vi "GetStaleFilesFromDisk.vi"(8 "error in (no error)":errorcluster, 10 "BacklogBatchSize":i32, 11 "data directory":path) -> (0 "error out":errorcluster, 2 "files found":i32, 3 "file paths":path[](array[path]))   [LabVIEW 2017, in "FileManager.lvlib"]
uses:
  <vilib>/addons/InsightCM/Devices/Shared/Common/FileManager/FileManager.lvlib
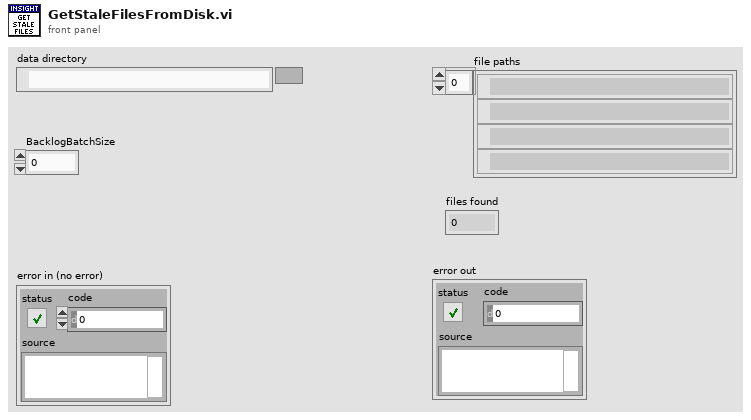
[diagram p1: front panel]
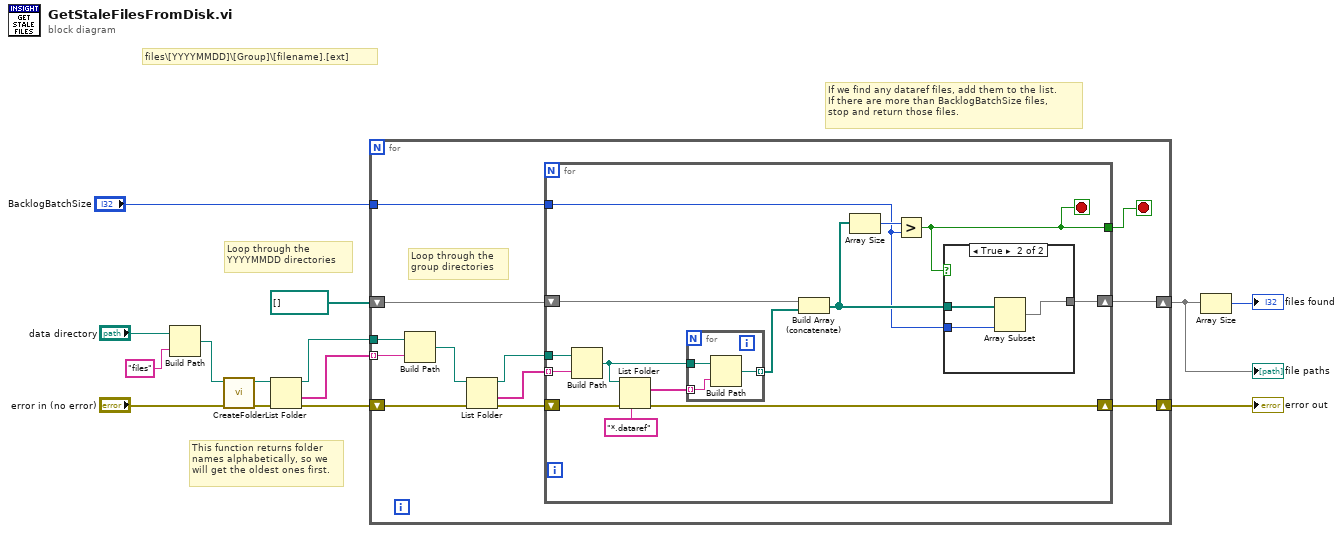
[diagram p0: block diagram]
diagram:
  # "If we find any dataref files, add them to the list.  \nIf there are more than BacklogBatchSize files,\nstop and return those files."
  # "files\\[YYYYMMDD]\\[Group]\\[filename].[ext]"
  # "This function returns folder\nnames alphabetically, so we \nwill get the oldest ones first."
  # "Loop through the \nYYYYMMDD directories"
  n1 = Build Path(base path="data directory", name or relative path="files") -> (appended path=w13:path)
  n2 = call <vilib>:"CreateFolder.vi"("error in (no error)"="error in (no error)", "folder"=w13) -> ("error out"=w10:errorcluster, "folder out"=w11:path)  [unwired: 8 in]
  n3 = List Folder(path=w11, error in=w10) -> (path out=w9:path, folder names=w7:string[], error out=w8:errorcluster)  [unwired: 3 out]
  n4 = for {
    tunnel: w7 -> [w26] mode=indexing
    tunnel: w9 -> [w25]
    shift-right: [w18] -> w6
    shift-left: w8 -> [w23]
    shift-right: [w16] -> w2
    shift-left: path[] [] ("file names") -> [w17]
    tunnel: "BacklogBatchSize" -> [w15]
    stop <- w19 stop-if-true
    # "Loop through the \ngroup directories"
    n5 = Build Path(base path=w25, name or relative path=w26) -> (appended path=w24:path)
    n6 = List Folder(path=w24, error in=w23) -> (path out=w21:path, folder names=w22:string[], error out=w20:errorcluster)  [unwired: 3 out]
    n7 = for {
      tunnel: w22 -> [w40] mode=indexing
      tunnel: w21 -> [w39]
      shift-right: [w36] -> w18
      shift-left: w20 -> [w35]
      tunnel: [w30] -> w19
      shift-right: [w28] -> w16
      shift-left: w17 -> [w33]
      tunnel: w15 -> [w27]
      stop <- w30 stop-if-true
      n8 = Build Path(base path=w39, name or relative path=w40) -> (appended path=w37:path)
      n9 = List Folder(path=w37, pattern="*.dataref", error in=w35) -> (filenames=w34:string[], error out=w36:errorcluster)  [unwired: 3 out]
      n10 = for {
        tunnel: w34 -> [w45] mode=indexing
        tunnel: w37 -> [w46]
        tunnel: [w47] -> w31 mode=indexing
        n11 = Build Path(base path=w46, name or relative path=w45) -> (appended path=w47:path)
      }
      n12 = Build Array (concatenate)(w33, w31) -> (w29:path[])
      n13 = Array Size(array=w29) -> (size(s)=w32:i32)
      n14 = Greater?(x=w32, y=w27) -> (0:w30:bool)
      n15 = case shown="True" w30 {
        tunnel: w29 -> [w41 w44]
        tunnel: w27 -> [_ w43]
        tunnel: [w41 w42] -> w28
        frame False {
        }
        frame True {
          n16 = Array Subset(array=w44, length=w43) -> (w42:path[])  [unwired: 1 in]
        }
      }
    }
  }
  "error out" <- w6
  "file paths" <- w2
  n17 = Array Size(array=w2) -> (size(s)=→"files found":i32)
